vi "Riffle.vi"   [LabVIEW 2020, in "NI_AALBase.lvlib"]
doc: "Riffles the elements in the input array <B>X</B>. Wire data to the <B>X</B> input to determine the polymorphic instance to use or manually select the instance."
uses:
  <vilib>/Analysis/NI_AALBase.lvlib
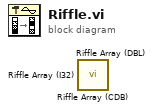
[diagram p0: block diagram]
diagram:
  n1 = call <vilib>:"Riffle Array (CDB).vi"() -> ()  [unwired: 9 in, 3 out]
  n2 = call <vilib>:"Riffle Array (DBL).vi"() -> ()  [unwired: 9 in, 3 out]
  n3 = call <vilib>:"Riffle Array (I32).vi"() -> ()  [unwired: 9 in, 3 out]
